vi "Data Updated.vi"(8 "error in (no error)":errorcluster, 9 "En MAP":u16, 10 "WiBCI16T Data in":T1 {"Reg Map"."ADS2" format="%x"; "Reg Map"."ADS1" format="%x"}) -> (0 "error out":errorcluster)   [LabVIEW 2016, in "Acquisition.lvlib"]
doc: "Broadcasts the latest data acquired\n_____\nCreated using Delacor QMH Event Scripter 4.0.0.65.\n_____\nBased on DQMH Project Template 6.1.0.94."
uses:
  Acquisition.lvlib
  WiBCI16T_Data.ctl
  WiBCI16T_Status.ctl
  Reg_Map.ctl
  Data Updated Argument--cluster.ctl
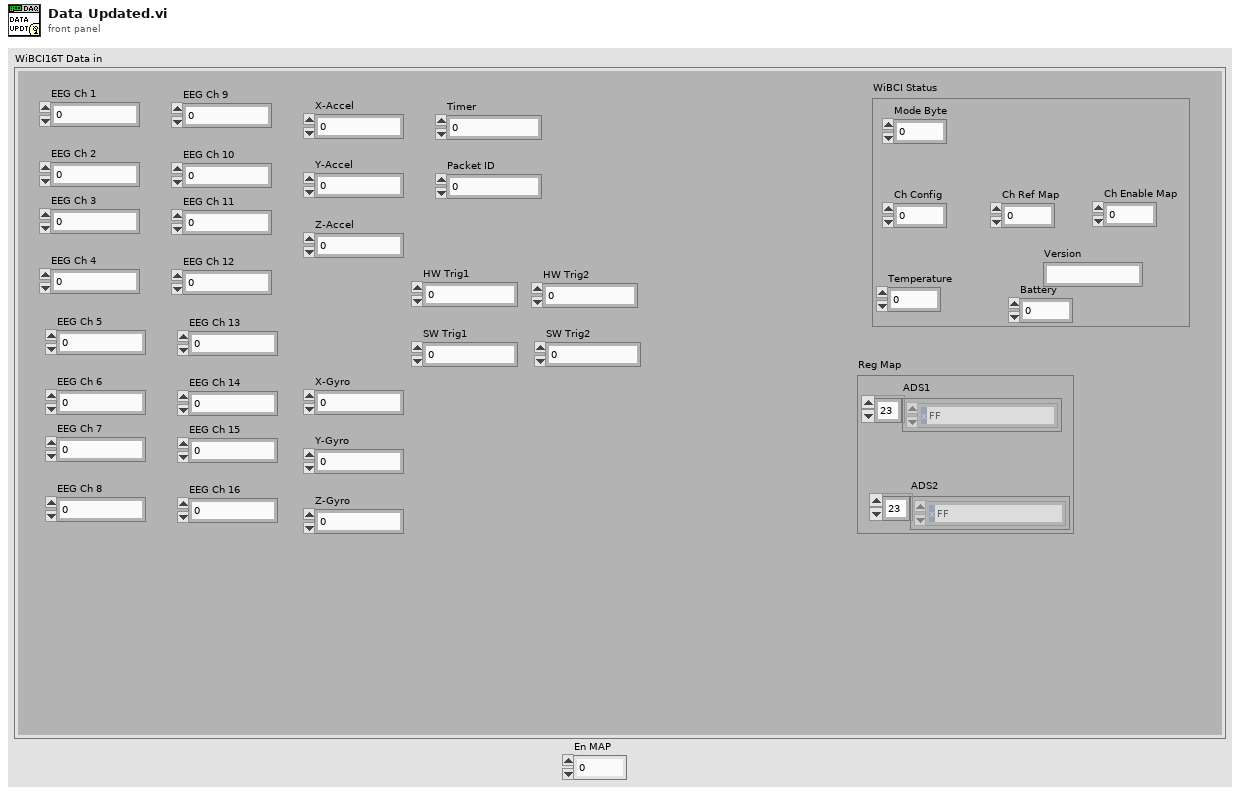
[diagram p1: front panel]
types:
  T1 = typedef "Acquisition.lvlib/WiBCI16T_Data.ctl" = cluster{"EEG Ch 1":dbl, "EEG Ch 2":dbl, "EEG Ch 3":dbl, "EEG Ch 4":dbl, "EEG Ch 5":dbl, "EEG Ch 6":dbl, "EEG Ch 7":dbl, "EEG Ch 8":dbl, "EEG Ch 9":dbl, "EEG Ch 10":dbl, "EEG Ch 11":dbl, "EEG Ch 12":dbl, "EEG Ch 13":dbl, "EEG Ch 14":dbl, "EEG Ch 15":dbl, "EEG Ch 16":dbl, "X-Accel":i16, "Y-Accel":i16, "Z-Accel":i16, "X-Gyro":i16, "Y-Gyro":i16, "Z-Gyro":i16, "Timer":u32, "Packet ID":u32, "HW Trig1":u8, "SW Trig1":i8, "HW Trig2":u8, "SW Trig2":i8, "WiBCI Status":T2, "Reg Map":T3}
  T2 = typedef "Acquisition.lvlib/WiBCI16T_Status.ctl" = cluster{"Mode Byte":u8, "Ch Config":u8, "Ch Ref Map":u16, "Ch Enable Map":u16, "Temperature":sgl, "Battery":u8, "Version":string}
  T3 = typedef "Acquisition.lvlib/Reg_Map.ctl" = cluster{"ADS1":u8[], "ADS2":u8[]}
  T4 = typedef "Acquisition.lvlib/Data Updated Argument--cluster.ctl" = cluster{"WiBCI16T Data out":T1, "En MAP":u16}
  T5 = typedef "Acquisition.lvlib/Broadcast Events--cluster.ctl" = cluster{"Module Did Init":refnum<user-event>, "Status Updated":refnum<user-event>, "Error Reported":refnum<user-event>, "Module Did Stop":refnum<user-event>, "Update Module Execution Status":refnum<user-event>, "Acquisition Started":refnum<user-event>, "Acquisition Stopped":refnum<user-event>, "Data Updated":refnum<user-event>, "Device Calibrated":refnum<user-event>, "Impedance Data Updated":refnum<user-event>, "CNV Data Updated":refnum<user-event>}
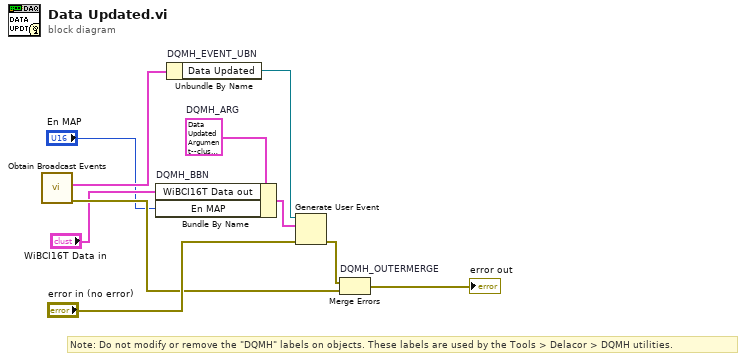
[diagram p0: block diagram]
diagram:
  w5 = T4 {"WiBCI16T Data out"={"EEG Ch 1"=0.0, "EEG Ch 2"=0.0, "EEG Ch 3"=0.0, "EEG Ch 4"=0.0, "EEG Ch 5"=0.0, "EEG Ch 6"=0.0, "EEG Ch 7"=0.0, "EEG Ch 8"=0.0, "EEG Ch 9"=0.0, "EEG Ch 10"=0.0, "EEG Ch 11"=0.0, "EEG Ch 12"=0.0, "EEG Ch 13"=0.0, "EEG Ch 14"=0.0, "EEG Ch 15"=0.0, "EEG Ch 16"=0.0, "X-Accel"=0, "Y-Accel"=0, "Z-Accel"=0, "X-Gyro"=0, "Y-Gyro"=0, "Z-Gyro"=0, "Timer"=0, "Packet ID"=0, "HW Trig1"=0, "SW Trig1"=0, "HW Trig2"=0, "SW Trig2"=0, "WiBCI Status"={"Mode Byte"=0, "Ch Config"=0, "Ch Ref Map"=0, "Ch Enable Map"=0, "Temperature"=0.0, "Battery"=0, "Version"=""}, "Reg Map"={"ADS1"=[], "ADS2"=[]}}, "En MAP"=0}  # DQMH_ARG
  # "Note: Do not modify or remove the \"DQMH\" labels on objects. These labels are used by the Tools > Delacor > DQMH utilities."
  n1 = call "Obtain Broadcast Events.vi"() -> ("error out"=w4:errorcluster, "Acquisition Broadcast Events"=w3:T5)  [unwired: 10 in]
  n2 = Bundle By Name "DQMH_BBN"(cluster=w5, "WiBCI16T Data out"="WiBCI16T Data in", "En MAP"="En MAP") -> (w8:T4)
  n3 = Unbundle By Name "DQMH_EVENT_UBN"(w3) -> ("Data Updated"=w7:refnum<user-event>)
  n4 = Generate User Event(user event=w7, event data cluster=w8, error in="error in (no error)") -> (error out=w6:errorcluster)  [unwired: 1 in, 1 out]
  n5 = Merge Errors "DQMH_OUTERMERGE"(w6, w4) -> (→"error out":errorcluster)
